vi "Derivative (multiple).vi"(8 "error in (no error)":errorcluster, 9 "Type":enum16{"dy/dx vs x", "dx/dy vs y"}(ring), 11 "XY-data":cluster{"X-array":dbl[], "Y-array":dbl[]}[](array[cluster]) {"Y-array" format="%.2p"; "X-array" format="%.2p"}) -> (0 "error out":errorcluster, 2 "Differential out":cluster{"X-array":dbl[], "Y-array":dbl[]}[](array[cluster]), 3 "XY-data out":cluster{"X-array":dbl[], "Y-array":dbl[]}[](array[cluster]) {"Y-array" format="%.2p"; "X-array" format="%.2p"})   [LabVIEW 2019, in "xy_utilities.lvlib"]
doc: "Performs numerical differentiation of <b>XY-data</b> using the finite difference method.\n\n<b>Interval</b> is the range over which the finite difference is calculated.\n<b>Interval Units</b> defines the units of the <b>Interval</b> to be the number of points or the same units as the x (or y) data\n<b>Type</b> specifies taking a derivative with respect to x or y.\n\nWire data to the data input to determine the polymorphic instance to use or manually select the instance."
uses:
  xy_utilities.lvlib
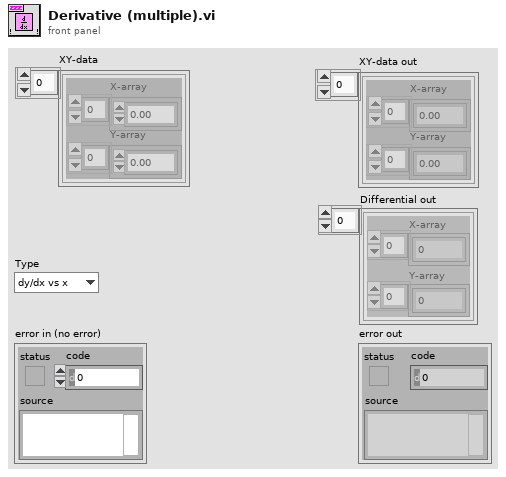
[diagram p1: front panel]
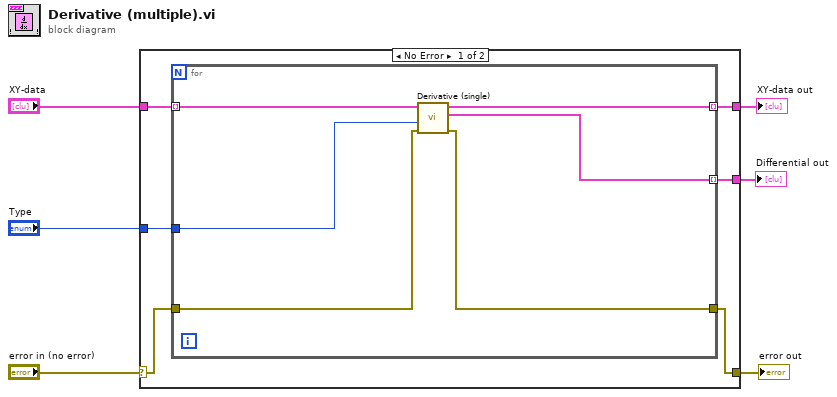
[diagram p0: block diagram]
diagram:
  n1 = case shown="No Error" "error in (no error)" {
    selector: "error in (no error)" -> [w10 w20]
    tunnel: [w9 w20] -> w5
    tunnel: "XY-data" -> [w12 w19]
    tunnel: [w11 w19] -> w3
    tunnel: "Type" -> [w8 _]
    tunnel: [w7 _] -> w1
    frame No Error {
      n2 = for {
        tunnel: w12 -> [w18] mode=indexing
        tunnel: [w17] -> w11 mode=indexing
        tunnel: w8 -> [w13]
        tunnel: [w16] -> w7 mode=indexing
        tunnel: w10 -> [w14]
        tunnel: [w15] -> w9
        n3 = call "Derivative (single).vi"("error in (no error)"=w14, "Type"=w13, "XY-data"=w18) -> ("error out"=w15:errorcluster, "Differential out"=w16:cluster{"X-array":dbl[], "Y-array":dbl[]}, "XY-data out"=w17:cluster{"X-array":dbl[], "Y-array":dbl[]})  [unwired: 6 in]
      }
    }
    frame Error {
    }
  }
  "error out" <- w5
  "XY-data out" <- w3
  "Differential out" <- w1
